vi "Start.vi"() -> ()   [LabVIEW 2023]
uses:
  8d223fd8-e801-47c5-b941-cb57a943469c.vi
  LV-Argparse/LV Argument Parser/Get.vi
  LV-Argparse/LV Argument Parser/LV Argument Parser.lvclass
panel:
  out "error out":errorcluster
  out "Message":string
  out "Data":map{string, variant[]}(c390)
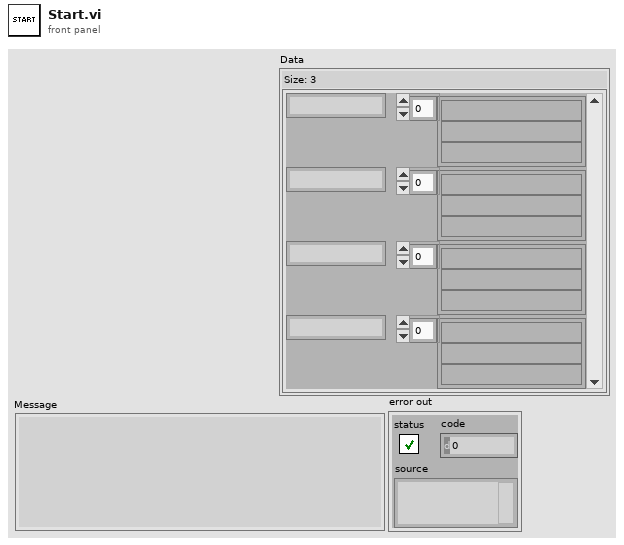
[diagram p1: front panel]
types:
  T1 = enum32{"Invalid", "Standard", "Closed", "Hidden", "Minimized", "Maximized"}
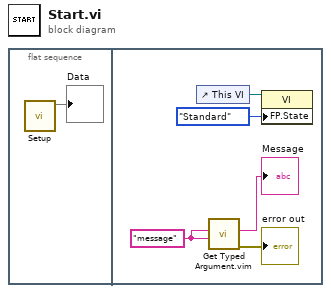
[diagram p0: block diagram]
diagram:
  n1 = flat-sequence {
    frame #0 {
      n2 = call "Setup.vi"() -> ("Data"=→"Data":map{string, variant[]})  [unwired: 11 in]
    }
    frame #1 {
      w2 = "message" ("Name")
      n3 = control-ref of="This VI"() -> (w6:refnum<vi>)
      n4 = call "Get Typed Argument.vim"("Name"=w2, "Type / Default"=w2) -> ("error out"=→"error out":errorcluster, "data"=→"Message":string)  [unwired: 7 in, 1 out]
      n5 = property class="VI"(reference=w6, "FP.State"=T1."Standard" ("Front Panel Window:State")) -> ()  [unwired: 1 in, 2 out]
    }
  }
